vi "Forward to Caller.vi"(8 "error in (no error)":errorcluster, 10 "Publisher Message":refnum<class "Publisher Msg.lvclass">, 11 "Actor in":refnum<class "Actor.lvclass">) -> (0 "error out":errorcluster, 3 "Actor out":refnum<class "Actor.lvclass">)   [LabVIEW 2020, in "Publisher.lvlib" / "Publisher.lvclass"]
doc: "Forward the publisher message to the caller."
uses:
  Publisher.lvclass
  PPL/HDH.Actor Framework.Core.Actor.lvlibp/1abvi3w/vi.lib/ActorFramework/Actor/Actor.lvclass
  Publisher Messages/Publisher Msg/Publisher Msg.lvclass
  Publisher Messages/Publisher Msg/Publisher Msg.lvclass/Publisher Msg.ctl
  PPL/HDH.Actor Framework.Core.Actor.lvlibp/1abvi3w/vi.lib/ActorFramework/Message Enqueuer/Message Enqueuer.lvclass
  C:/Current projects/WS/PPL/HDH.Actor Framework.Core.Actor.lvlibp/1abvi3w/vi.lib/ActorFramework/Message/Message.lvclass
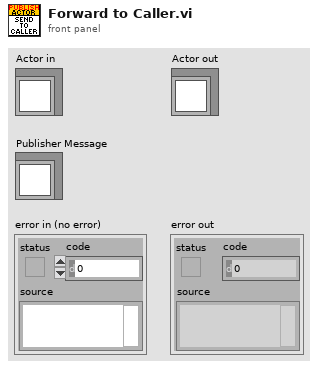
[diagram p1: front panel]
types:
  T1 = typedef "HDH.Actor Framework.Core.Actor.lvlibp/Message Enqueuer.lvclass/Message Priority.ctl" = enum16{"Low", "Normal", "High"}
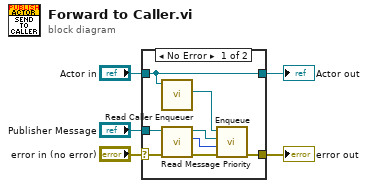
[diagram p0: block diagram]
diagram:
  n1 = case shown="No Error" "error in (no error)" {
    selector: "error in (no error)" -> [w7 w15]
    tunnel: [w11 w15] -> w4
    tunnel: [w13 w14] -> w2
    tunnel: "Actor in" -> [w13 w14]
    tunnel: "Publisher Message" -> [w10 _]
    frame No Error {
      n2 = call "Read Caller Enqueuer.vi"("Actor"=w13) -> ("Caller Enqueuer"=w12:refnum<class "Message Enqueuer.lvclass">)  [unwired: 10 in]
      n3 = call "Read Message Priority.vi"("error in (no error)"=w7, "Publisher Msg in"=w10) -> ("error out"=w6:errorcluster, "Message Priority"=w8:T1, "Publisher Msg out"=w9:refnum<class "Publisher Msg.lvclass">)  [unwired: 7 in]
      n4 = call "Enqueue.vi"("error in (no error)"=w6, "Message Priority (Normal)"=w8, "Message"=w9, "Message Enqueuer in"=w12) -> ("error out"=w11:errorcluster)  [unwired: 6 in, 1 out]
    }
    frame Error {
    }
  }
  "error out" <- w4
  "Actor out" <- w2
